vi "set_Directories.vi"(0 "Host_Reference":refnum<class "HGF_Reference.lvclass">, 2 "timeout in ms (-1)":i32=-1, 5 "error in (no error)":errorcluster) -> (14 "dup Host_Reference":refnum<class "HGF_Reference.lvclass">, 19 "error out":errorcluster)   [LabVIEW 2009, in "MoAgSy.lvlib" / "MoAgSy_Host.lvclass"]
doc: "<B>public</B> VI sets local directories of referenced Host.\n<B>Vi frontpanel has to be shown at vi call.</B>\n\nF.Berck@gsi.de\nGSI Darmstadt 2009"
uses:
  MoAgSy_Host.lvclass
  HGF_BaseClasses/HGF_Reference/HGF_Reference.lvclass
panel:
  in  "Directories":T1
  in  "Cancel":bool
  in  "Apply":bool
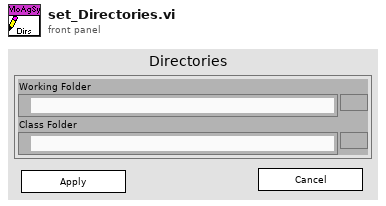
[diagram p1: front panel]
types:
  T1 = cluster{"Working Folder":path, "Class Folder":path}
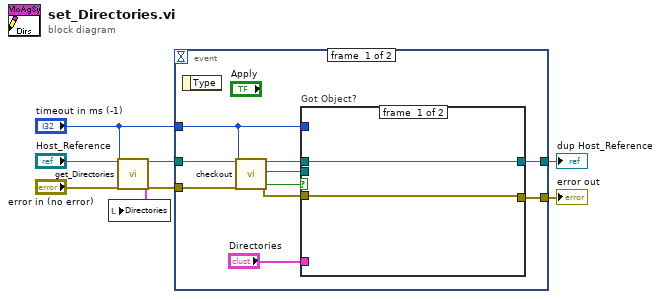
[diagram p0: block diagram]
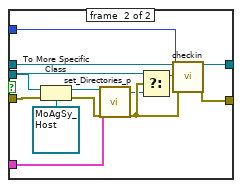
[diagram p2: hidden frame]
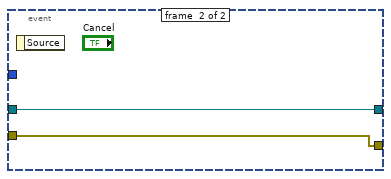
[diagram p3: hidden frame]
diagram:
  n1 = call "get_Directories.vi"("Host_Reference"="Host_Reference", "timeout in ms (-1)"="timeout in ms (-1)", "error in (no error)"="error in (no error)") -> ("dup Host_Reference"=w5:refnum<class "HGF_Reference.lvclass">, "Directories"=w1:T1, "error out"=w2:errorcluster)  [unwired: 14 out]
  n2 = local write "Directories"(w1) -> ()
  n3 = event shown="[1] \"Cancel\": Value Change;  Panel Close" {
    selector: _ -> [_ _]
    dyn-events: _ -> [_ _]
    timeout: _ -> [_ _]
    tunnel: [w18 w34] -> w7
    tunnel: [w17 w35] -> w8
    tunnel: "timeout in ms (-1)" -> [w13 _]
    tunnel: w5 -> [w12 w35]
    tunnel: w2 -> [w11 w34]
    event #0 {
      n4 = event-data() -> ()  [unwired: 2 out]
      n5 = call "checkout.vi"("HGF_Reference"=w12, "timeout in ms (-1)"=w13, "error in (no error)"=w11) -> ("dup HGF_Reference"=w16:refnum<class "HGF_Reference.lvclass">, "Object"=w14:refnum<class>, "got object?"=w15:bool, "error out"=w10:errorcluster)  [unwired: 13 out]
      n6 = case "Got Object?" shown="True" w15 {
        tunnel: w14 -> [_ w22]
        tunnel: w16 -> [w20 w31]
        tunnel: [w20 w30] -> w17
        tunnel: w13 -> [_ w29]
        tunnel: [w19 w28] -> w18
        tunnel: w10 -> [w19 w27]
        tunnel: "Directories" -> [_ w24]
        frame #0 {
        }
        frame #1 {
          n7 = To More Specific Class(target class=refnum<class "MoAgSy_Host.lvclass"> refnum ("MoAgSy.lvlib:MoAgSy_Host.lvclass"), reference=w22, error in=w27) -> (specific class reference=w26:refnum<class "MoAgSy_Host.lvclass">, error out=w25:errorcluster)
          n8 = call "set_Directories_p.vi"("MoAgSy_Host"=w26, "Directories"=w24, "error in (no error)"=w25) -> ("dup MoAgSy_Host"=w23:refnum<class "MoAgSy_Host.lvclass">, "error out"=w33:errorcluster)  [unwired: 15 out]
          n9 = Select(t=w22, s=w33, f=w23) -> (s? t:f=w21:refnum<class>)
          n10 = call "checkin.vi"("HGF_Reference"=w31, "Object"=w21, "timeout /ms (-1)"=w29, "error in (no error)"=w33) -> ("dup HGF_Reference"=w30:refnum<class "HGF_Reference.lvclass">, "error out"=w28:errorcluster)  [unwired: 14 out]
        }
      }
    }
    event #1 {
      n11 = event-data() -> ()  [unwired: 2 out]
    }
  }
  "dup Host_Reference" <- w8
  "error out" <- w7
